vi "New Service Dialog.vi"() -> (2 "Create New":bool, 3 "Service Details":T1)   [LabVIEW 2016, in "Assert Display.lvlib" / "Service Config Display.lvlib" / "Service Config Display.lvclass"]
doc: "Pop up dialog to ask the user for details of a new alias"
uses:
  Service Config Display.lvclass
  Service Details.ctl
  Assert Display/Assert Display.lvlib
panel:
  in  "OK":bool
  in  "IP Address":string(combo)
  in  "Name":string
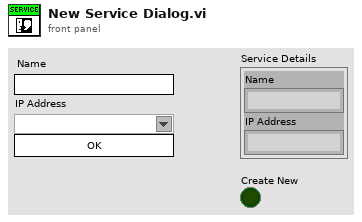
[diagram p1: front panel]
types:
  T1 = typedef "Assert Display.lvlib/Service Details.ctl" = cluster{"Name":string, "IP Address":string}
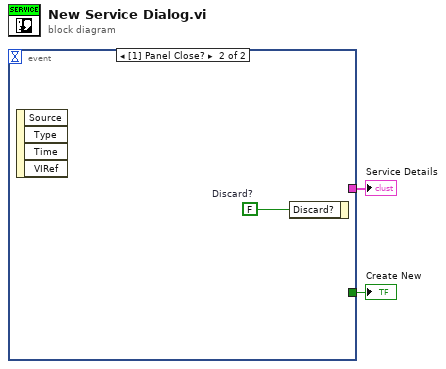
[diagram p0: block diagram]
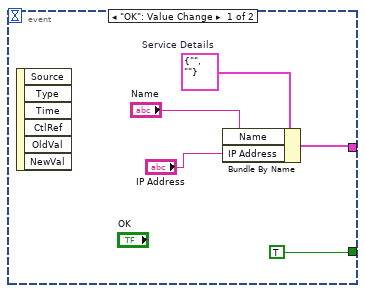
[diagram p2: hidden frame]
diagram:
  n1 = event shown="[1] Panel Close?" {
    selector: _ -> [_ _]
    dyn-events: _ -> [_ _]
    timeout: _ -> [_ _]
    tunnel: [w4 _] -> w2
    tunnel: [TRUE _] -> w1
    event "OK": Value Change {
      w5 = T1 {"Name"="", "IP Address"=""}  # Service Details
      n2 = event-data() -> ()  [unwired: 1 in, 6 out]
      n3 = Bundle By Name(cluster=w5, "Name"="Name", "IP Address"="IP Address") -> (w4:T1)
    }
    event Panel Close? {
      w8 = FALSE  # Discard?
      n4 = event-data() -> ()  [unwired: 1 in, 4 out]
      n5 = event-data("Discard?"=w8) -> ()  [unwired: 1 in, 1 out]
    }
  }
  "Service Details" <- w2
  "Create New" <- w1
